vi "filterToBool.vi"(6 "AVG Filter type":T2, 8 "error in (no error)":errorcluster, 9 "MedianFilter":T1, 10 "Filter":T1, 11 "Electrometer in":refnum<class "Electrometer.lvclass">) -> (0 "error out":errorcluster, 1 "MedianFilter":bool, 2 "Filter":bool, 3 "Electrometer out":refnum<class "Electrometer.lvclass">, 4 "AVG Filter type":bool)   [LabVIEW 2016, in "Electrometer.lvclass"]
uses:
  Electrometer.lvclass
  MED Filter Type.ctl
  AVG Filter type.ctl
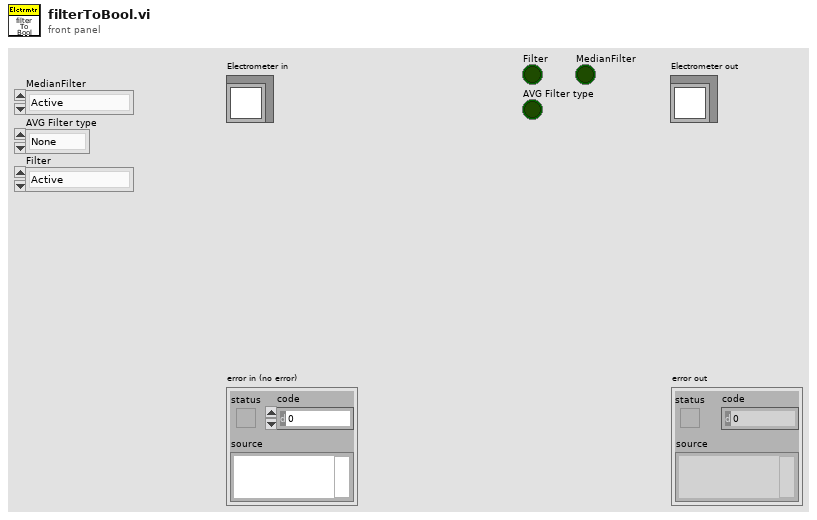
[diagram p1: front panel]
types:
  T1 = typedef "Electrometer.lvclass/MED Filter Type.ctl" = enum16{"Active", "None"}
  T2 = typedef "Electrometer.lvclass/AVG Filter type.ctl" = enum16{"None", "Scalar", "Advanced"}
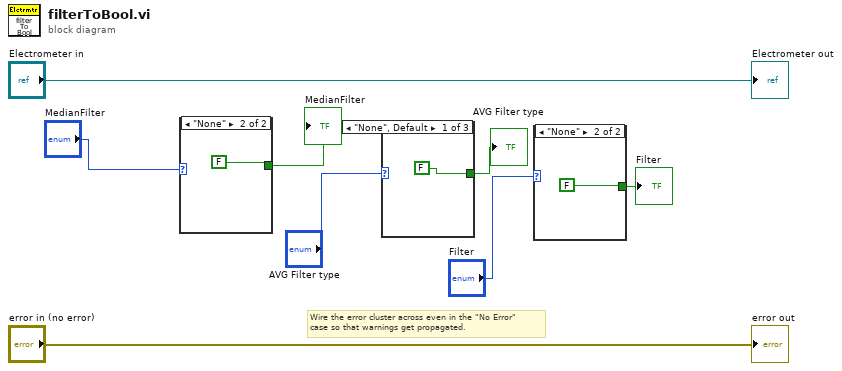
[diagram p0: block diagram]
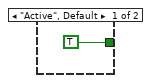
[diagram p2: hidden frame]
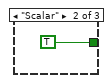
[diagram p3: hidden frame]
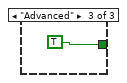
[diagram p4: hidden frame]
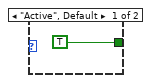
[diagram p5: hidden frame]
diagram:
  # "Wire the error cluster across even in the \"No Error\"\ncase so that warnings get propagated."
  n1 = case shown="\"None\"" "MedianFilter" {
    tunnel: [TRUE FALSE] -> w1
    frame "Active", Default {
    }
    frame "None" {
    }
  }
  "MedianFilter" <- w1
  n2 = case shown="\"None\", Default" "AVG Filter type" {
    tunnel: [FALSE TRUE TRUE] -> w2
    frame "None", Default {
    }
    frame "Scalar" {
    }
    frame "Advanced" {
    }
  }
  "AVG Filter type" <- w2
  n3 = case shown="\"None\"" "Filter" {
    tunnel: [TRUE FALSE] -> w3
    frame "Active", Default {
    }
    frame "None" {
    }
  }
  "Filter" <- w3
  "error out" <- "error in (no error)"
  "Electrometer out" <- "Electrometer in"
